vi "Disable_Enable_Controls.vi"(0 "Gray_Out_Control":refnum<vi>[](array[refnum]), 5 "Enable_Control":refnum<vi>[](array[refnum]), 7 "Disable_Control":refnum<vi>[](array[refnum]), 11 "Error_In":errorcluster) -> (15 "Error_Out":errorcluster)   [LabVIEW 2021]
doc: "Used to disable and enable the controls"
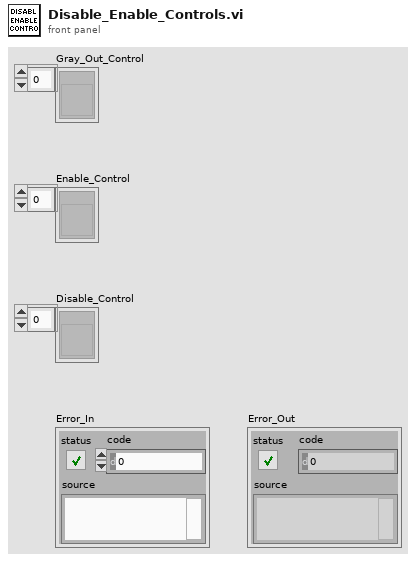
[diagram p1: front panel]
types:
  T1 = enum8{"Enabled", "Disabled", "Disabled and Grayed Out"}
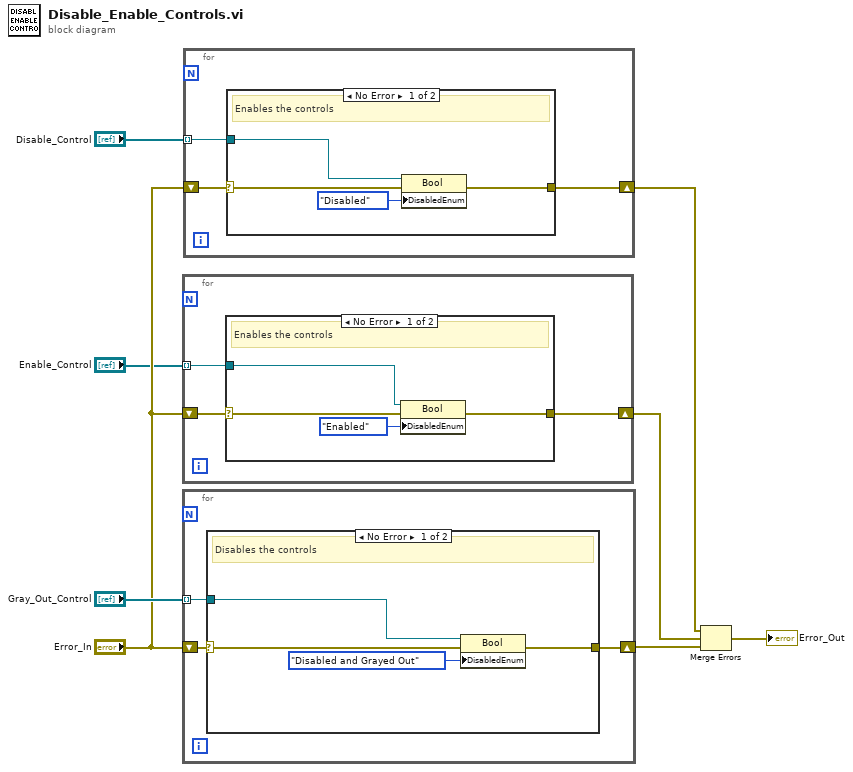
[diagram p0: block diagram]
diagram:
  n1 = for {
    shift-right: [w11] -> w5
    shift-left: "Error_In" -> [w10]
    tunnel: "Enable_Control" -> [w9] mode=indexing
    n2 = case shown="No Error" w10 {
      selector: w10 -> [w13 w16]
      tunnel: [w15 w16] -> w11
      tunnel: w9 -> [w12 _]
      frame No Error {
        # "Enables the controls"
        n3 = property class="Bool"(reference=w12, error in=w13, "DisabledEnum"=T1."Enabled" ("Disabled")) -> (error out=w15:errorcluster)  [unwired: 1 out]
      }
      frame Error {
      }
    }
  }
  n4 = for {
    shift-right: [w19] -> w7
    shift-left: "Error_In" -> [w17]
    tunnel: "Gray_Out_Control" -> [w18] mode=indexing
    n5 = case shown="No Error" w17 {
      selector: w17 -> [w20 w24]
      tunnel: [w23 w24] -> w19
      tunnel: w18 -> [w22 _]
      frame No Error {
        # "Disables the controls"
        n6 = property class="Bool"(reference=w22, error in=w20, "DisabledEnum"=T1."Disabled and Grayed Out" ("Disabled")) -> (error out=w23:errorcluster)  [unwired: 1 out]
      }
      frame Error {
      }
    }
  }
  n7 = for {
    shift-right: [w27] -> w4
    shift-left: "Error_In" -> [w25]
    tunnel: "Disable_Control" -> [w26] mode=indexing
    n8 = case shown="No Error" w25 {
      selector: w25 -> [w28 w32]
      tunnel: [w31 w32] -> w27
      tunnel: w26 -> [w30 _]
      frame No Error {
        # "Enables the controls"
        n9 = property class="Bool"(reference=w30, error in=w28, "DisabledEnum"=T1."Disabled" ("Disabled")) -> (error out=w31:errorcluster)  [unwired: 1 out]
      }
      frame Error {
      }
    }
  }
  n10 = Merge Errors(w4, w5, w7) -> (→"Error_Out":errorcluster)
